vi "Get Paths.vi"() -> (1 "Source Folder":path, 3 "Template Folder":path)   [LabVIEW 2020, in "ADAS_IO_Template_MDO.lvclass"]
uses:
  ADAS_IO_Template_MDO.lvclass
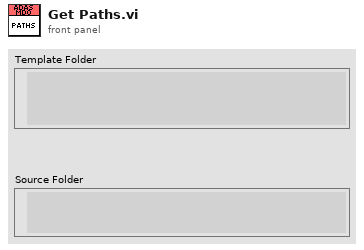
[diagram p1: front panel]
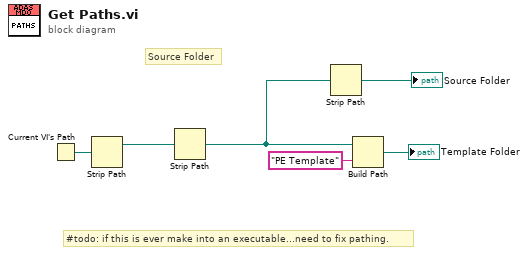
[diagram p0: block diagram]
diagram:
  # "#todo: if this is ever make into an executable...need to fix pathing."
  # "Source Folder"
  n1 = Current VI's Path() -> (path=w3:path)
  n2 = Strip Path(path=w3) -> (stripped path=w4:path)  [unwired: 1 out]
  n3 = Strip Path(path=w4) -> (stripped path=w2:path)  [unwired: 1 out]
  n4 = Strip Path(path=w2) -> (stripped path=→"Source Folder":path)  [unwired: 1 out]
  n5 = Build Path(base path=w2, name or relative path="PE Template") -> (appended path=→"Template Folder":path)
